vi "sub_ekf_covariance-ellipse.vi"() -> ()   [LabVIEW 2019]
uses:
  <vilib>/Analysis/Matrix/Datatypes/RealMatrix.ctl
  <vilib>/Analysis/7linalg.llb/Real Eigenvalues and Vectors.vi
  <vilib>/Analysis/NI_AALPro.lvlib
  <vilib>/Analysis/Matrix/NI_Matrix.lvlib
panel:
  out "b":dbl
  out "a":dbl
  out "Eigenvalues":cdb[](array[numeric]) caption="고유값"
  out "smallind":dbl
  out "bigind":dbl=1.0
  out "Pxy":T1
  in  "PEst":T1
  in  "xEst":T1
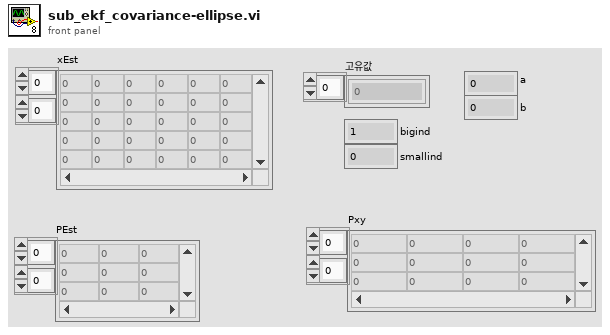
[diagram p1: front panel]
types:
  T1 = typedef "NI_Matrix.lvlib/RealMatrix.ctl" = dbl[][]
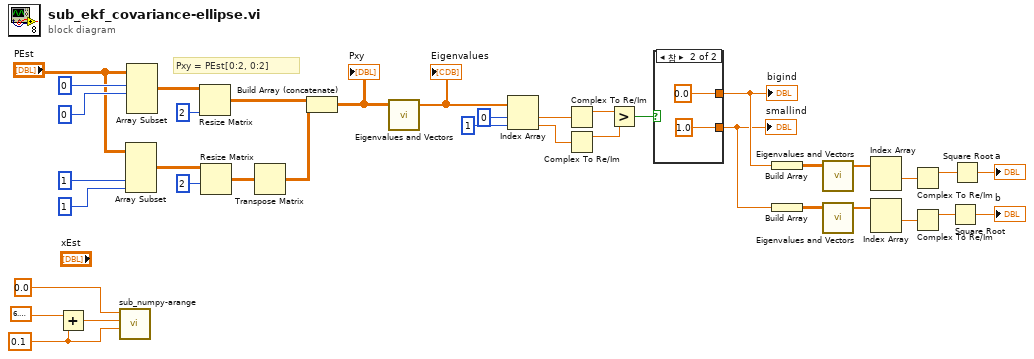
[diagram p0: block diagram]
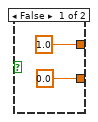
[diagram p2: hidden frame]
diagram:
  w14 = 0.1 ("y")
  # "Pxy = PEst[0:2, 0:2]"
  n1 = Add(x=6.283185307179586, y=w14) -> (x+y=w15:dbl)
  n2 = call "sub_numpy-arange.vi"("step"=w14, "max"=w15, "start"=0.0) -> ()  [unwired: 8 in, 1 out]
  n3 = Array Subset(array="PEst", index (col)=1 ("열 1"), length (col)=1 ("열 N")) -> (w31:T1)  [unwired: 2 in]
  n4 = Array Subset(array="PEst", index (row)=0 ("행 1"), length (row)=0 ("행 N")) -> (w34:T1)  [unwired: 2 in]
  n5 = Resize Matrix(1:2 ("열의 개수"), 4:w34) -> (0:w29:T1)  [unwired: 1 in]
  n6 = Resize Matrix(2:2 ("행의 개수"), 4:w31) -> (0:w28:T1)  [unwired: 1 in]
  n7 = Transpose Matrix(1:w28) -> (0:w27:T1)
  n8 = Build Array (concatenate)(w29, w27) -> (w26:T1)
  "Pxy" <- w26
  n9 = call-poly <vilib>:"Eigenvalues and Vectors.vi"("Input Matrix"=w26) -> ("Eigenvalues"=w25:cdb[])  [unwired: 2 in, 2 out]
  "Eigenvalues" <- w25
  n10 = Index Array(array=w25, index #1=0 ("인덱스"), index #2=1 ("인덱스")) -> (element #1=w22:cdb, element #2=w21:cdb)
  n11 = Complex To Re/Im(x + iy=w22) -> (x=w19:dbl)  [unwired: 1 out]
  n12 = Complex To Re/Im(x + iy=w21) -> (x=w20:dbl)  [unwired: 1 out]
  n13 = Greater?(x=w19, y=w20) -> (0:w18:bool)
  n14 = case shown="참" w18 {
    tunnel: [1.0 0.0] -> w13
    tunnel: [0.0 1.0] -> w10
    frame False {
    }
    frame True {
    }
  }
  "bigind" <- w13
  "smallind" <- w10
  n15 = Build Array(w13) -> (w12:T1)
  n16 = Build Array(w10) -> (w11:T1)
  n17 = call-poly <vilib>:"Eigenvalues and Vectors.vi"("Input Matrix"=w12) -> ("Eigenvalues"=w8:cdb[])  [unwired: 2 in, 2 out]
  n18 = call-poly <vilib>:"Eigenvalues and Vectors.vi"("Input Matrix"=w11) -> ("Eigenvalues"=w6:cdb[])  [unwired: 2 in, 2 out]
  n19 = Index Array(array=w8) -> (element #1=w9:cdb)  [unwired: 2 in, 1 out]
  n20 = Index Array(array=w6) -> (element #1=w7:cdb)  [unwired: 2 in, 1 out]
  n21 = Complex To Re/Im(x + iy=w9) -> (x=w5:dbl)  [unwired: 1 out]
  n22 = Complex To Re/Im(x + iy=w7) -> (x=w3:dbl)  [unwired: 1 out]
  n23 = Square Root(x=w3) -> (sqrt(x)=→"b":dbl)
  n24 = Square Root(x=w5) -> (sqrt(x)=→"a":dbl)
